vi "Initial Target.vi"(1 "Initial Position":T2[](array[typedef])) -> (0 "Initial Target":T1[](array[typedef]))   [LabVIEW 2009]
uses:
  Control Loop/Act & Cart Commands.ctl
  Target Data.ctl
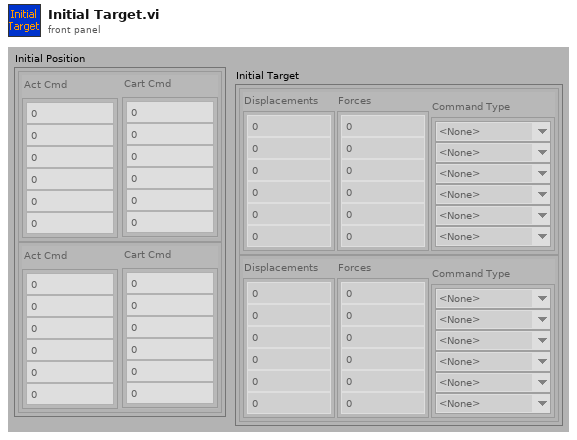
[diagram p1: front panel]
types:
  T1 = typedef "Target Data.ctl" = cluster{"Displacements":dbl[], "Command Type":enum16{"<None>", "Displacement", "Force"}[], "Forces":dbl[]}
  T2 = typedef "Act & Cart Commands.ctl" = cluster{"Act Cmd":dbl[], "Cart Cmd":dbl[]}
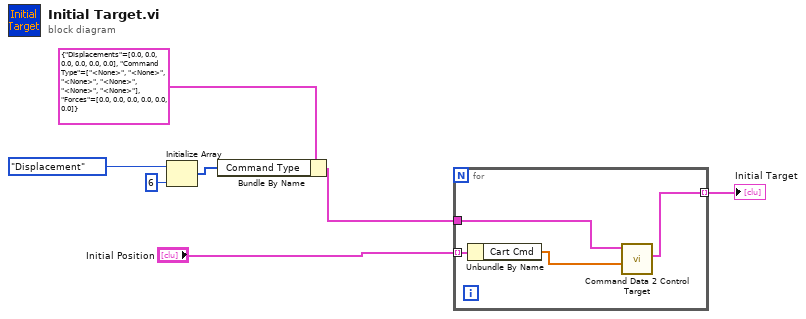
[diagram p0: block diagram]
diagram:
  n1 = Initialize Array(enum16{"<None>", "Displacement", "Force"}."Displacement" ("Enum"), 6 ("dimension size")) -> (w2:enum16{"<None>", "Displacement", "Force"}[])
  n2 = Bundle By Name(cluster=T1 {"Displacements"=[0.0, 0.0, 0.0, 0.0, 0.0, 0.0], "Command Type"=[enum."<None>", enum."<None>", enum."<None>", enum."<None>", enum."<None>", enum."<None>"], "Forces"=[0.0, 0.0, 0.0, 0.0, 0.0, 0.0]} ("Current Target"), "Command Type"=w2) -> (w1:T1)
  n3 = for {
    tunnel: [w11] -> w6 mode=indexing
    tunnel: "Initial Position" -> [w10] mode=indexing
    tunnel: w1 -> [w9]
    n4 = Unbundle By Name(w10) -> ("Cart Cmd"=w8:dbl[])
    n5 = call "Command Data 2 Control Target.vi"("Current Command"=w8, "Current Target"=w9) -> ("Output"=w11:T1)  [unwired: 9 in]
  }
  "Initial Target" <- w6
